vi "测试-二维数组转为一维数组.vi"() -> ()   [LabVIEW 2018]
panel:
  out "元素":dbl[](array[numeric])
  in  "原有的二维数组":dbl[][](array[numeric])=[[0.0, 1.0, 2.0, 3.0], [4.0, 5.0, 6.0, 7.0], [8.0, 9.0, 10.0, 11.0], [12.0, 13.0, 14.0, 15.0]] format="%#.6g"
  # "参考来源：https://lavag.org/topic/2423-how-to-send-2d-array-into-1d-array/"
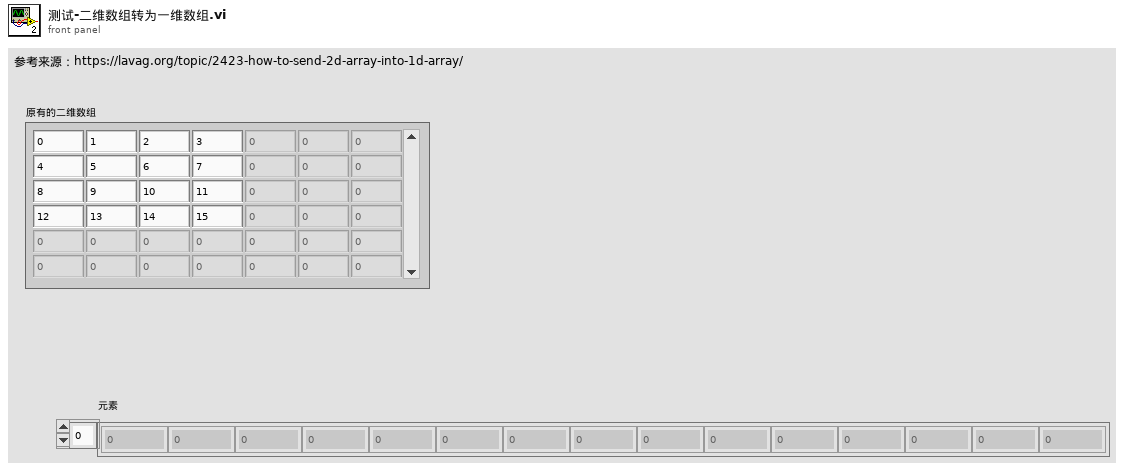
[diagram p1: front panel]
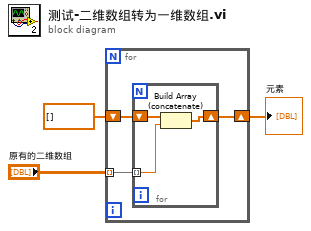
[diagram p0: block diagram]
diagram:
  n1 = for {
    tunnel: "原有的二维数组" -> [w6] mode=indexing
    shift-right: [w4] -> w1
    shift-left: dbl[] [] ("元素") -> [w5]
    n2 = for {
      tunnel: w6 -> [w9] mode=indexing
      shift-right: [w7] -> w4
      shift-left: w5 -> [w8]
      n3 = Build Array (concatenate)(w8, w9) -> (w7:dbl[])
    }
  }
  "元素" <- w1
